vi "CR-字符检测参数读取.vi"(7 "error in (no error)":errorcluster caption="错误输入（无错误）", 10 "基路径":path) -> (0 "error out":errorcluster caption="错误输出", 1 "字符识别参数":T5={"Parameters (OCR/OCV 1)"={"Threshold Data"={"Method"=enum."Local", "Looking for"=1, "Color Mode"=0, "Kernel Size"={"Width"=32, "Height"=32}, "Ranges"=[{"Min"=1, "Max"=255}]}, "Reject Border"=TRUE, "Number Of Erosions"=0, "Size & Spacing"={"Segment Algorithm"=0, "Min Bounding Rect Width"=1, "Max Bounding Rect Width"=65536, "Min Bounding Rect Height"=1, "Max Bounding Rect Height"=65536, "Min Character Size"=20, "Max Character Size"=65536, "Min Char Spacing"=1, "Max Horiz Element Spacing"=1, "Max Vert Element Spacing"=0, "Max Space Distance"=65536}, "Read Options"={"Read Strategy"=1, "Read Resolution"=2, "Scale Dependant"=FALSE, "Aspect Ratio"=400, "Acceptance Level"=700, "Substitution Character"="?", "MultiLine"=TRUE}, "Valid Characters"=[], "Use Text Pattern"=FALSE, "Orientation"=0, "# Lines Expected"=0, "Number of Blocks"=4}, "Rectangle"={"Left"=0, "Top"=0, "Right"=0, "Bottom"=0, "Rotation"=0.0}, "字符长度判定"=0.0, "Reference System"={"Origin"={"X"=1245.2058, "Y"=1038.7815}, "Angle (deg)"=0.021420227, "Axis Reference"=0}, "File Path (字符库)"=path "D:/Inspect System/Source Code/Template Program/字符模板.abc", "File Path (连接件模板)"=path "D:/Inspect System/Source Code/Template Program/字符检测定位模板.png", "Url"="http://10.6.1.31:8080/MesInnerpackLineIO.asmx", "accessKey"="a45b2d3334ffs_\na45b2d3334ffs_"} {"Reference System"."Axis Reference" items=["Direct", "Indirect"]; "Rectangle"."Rotation" min=-90.0 max=90.0 step=1.0 format="%.2f"; "Rectangle"."Left" scale=0.0..1024.0; "Rectangle"."Right" scale=0.0..1024.0; "Parameters (OCR/OCV 1)"."Threshold Data"."Looking for" items=["Light on Dark", "Dark on Light"]; "Parameters (OCR/OCV 1)"."Threshold Data"."Color Mode" items=["RGB", "HSL", "HSV", "HSI"]; "Parameters (OCR/OCV 1)"."Size & Spacing"."Segment Algorithm" items=["None", "Shortest Segment", "Legacy Auto Split"]; "Parameters (OCR/OCV 1)"."Read Options"."Read Strategy" items=["Aggressive", "Conservative"]; "Parameters (OCR/OCV 1)"."Read Options"."Read Resolution" items=["Low", "Medium", "High"]; "Parameters (OCR/OCV 1)"."Valid Characters"."Pre-defined characters" items=["Any Character", "User-defined Characters", "Alphabetic", "Alphanumeric", "Uppercase Letters", "Lowercase Letters", "Decimal Digits", "Hexadecimal Digits", "Pattern", "Force Space"]; "Parameters (OCR/OCV 1)"."Orientation" items=["Baseline inside", "Baseline outside"]}, 2 "字符检测基础参数":T6={"IsNorImage"=TRUE, "Exposure Values"=100289, "ImagePath"=path "C:/Users/hedongpo/Desktop/514-hdp/Alignment Assemble System/Test Picture/B/3.bmp"} caption="参数界面" {"Exposure Values" scale=0.0..200000.0}, 3 "CR-CCD1字符定位参数":T4={"Rectangle"={"Left"=0, "Top"=0, "Right"=0, "Bottom"=0, "Rotation"=0.0}, "Settings"={"Curve Parameters"={"Extraction Mode"=0, "Edge Threshold"=35, "Edge Filter Size"=1, "Min Length"=25, "Row Search Step Size"=15, "Col Search Step Size"=15, "Max Endpoint Gap"=10, "Closed"=FALSE, "Subpixel"=FALSE}, "Match Mode"={"Rotation"=TRUE, "Scale"=FALSE, "Occlusion"=TRUE, "Reserved 1"=FALSE, "Reserved 2"=FALSE, "Reserved 3"=FALSE}, "Range Settings"=[{"Match Constraints"=0, "Min"=-17.0, "Max"=17.0}, {"Match Constraints"=2, "Min"=0.0, "Max"=25.0}], "Number of Matches"=1, "Minimum Match Score"=400.0, "SubPixel Accuracy"=FALSE, "Adv. Geometric Match Options 2"=[{"Setup Data Item"=21, "Item Value"=0.0}, {"Setup Data Item"=22, "Item Value"=1.0}]}, "Template File Path"=path "F:/Inspect System -2/Source Code/Template Program/程序1/字符定位模板.png"} {"Settings"."Curve Parameters"."Extraction Mode" items=["Normal", "Uniform Regions"]; "Settings"."Curve Parameters"."Edge Filter Size" items=["Fine", "Normal", "Contour Tracing"]; "Settings"."Curve Parameters"."Max Endpoint Gap" min=0; "Settings"."Curve Parameters"."Col Search Step Size" min=1 max=255 step=1; "Settings"."Curve Parameters"."Row Search Step Size" min=1 max=255 step=1; "Settings"."Curve Parameters"."Min Length" min=0; "Settings"."Curve Parameters"."Edge Threshold" min=1 max=350 step=1; "Settings"."Range Settings"."Max" format="%.2f"; "Settings"."Range Settings"."Min" format="%.2f"; "Settings"."Range Settings"."Match Constraints" items=["Rotation Angle (degrees)", "Scale Factor (%)", "Occlusion (%)"]; "Settings"."Adv. Geometric Match Options 2"."Setup Data Item" items=["Curve Extraction Mode", "Curve Edge Threshold", "Curve Edge Filter Size", "Min Curve Length", "Curve Row Search Step Size", "Curve Col Search Step Size", "Curve Max Endpoint Gap", "Extract Closed Curves", "Enable Subpixel Curve Extraction", "Enable Correlation Score", "Enable Subpixel Accuracy", "Subpixel Iterations", "Subpixel Tolerance", "Initial Match List Length", "Enable Target Template Curve Score", "Min Match Separation Distance", "Min Match Separation Angle", "Min Match Separation Scale", "Max Match Overlap", "Enable Coarse Result", "Enable Calibration Support", "Enable Contrast Reversal", "Search Strategy", "Refinement Match Factor", "Subpixel Match Factor"]; "Rectangle"."Rotation" format="%.2f"; "Rectangle"."Left" scale=0.0..1024.0; "Rectangle"."Right" scale=0.0..1024.0})   [LabVIEW 2017]
uses:
  <vilib>/vision/Pattern Matching.llb/IMAQ Curve Parameters.ctl
  <vilib>/vision/Pattern Matching.llb/IMAQ Match Range Setting.ctl
  <vilib>/Utility/xml.llb/Read From XML File(string).vi
  Global System.vi
panel:
  # "UI电源线反面标签1基础参数"
  # "D:\\Inspect System\\Source Code\\Template Program\\BlackTemplete"
  # "Range"
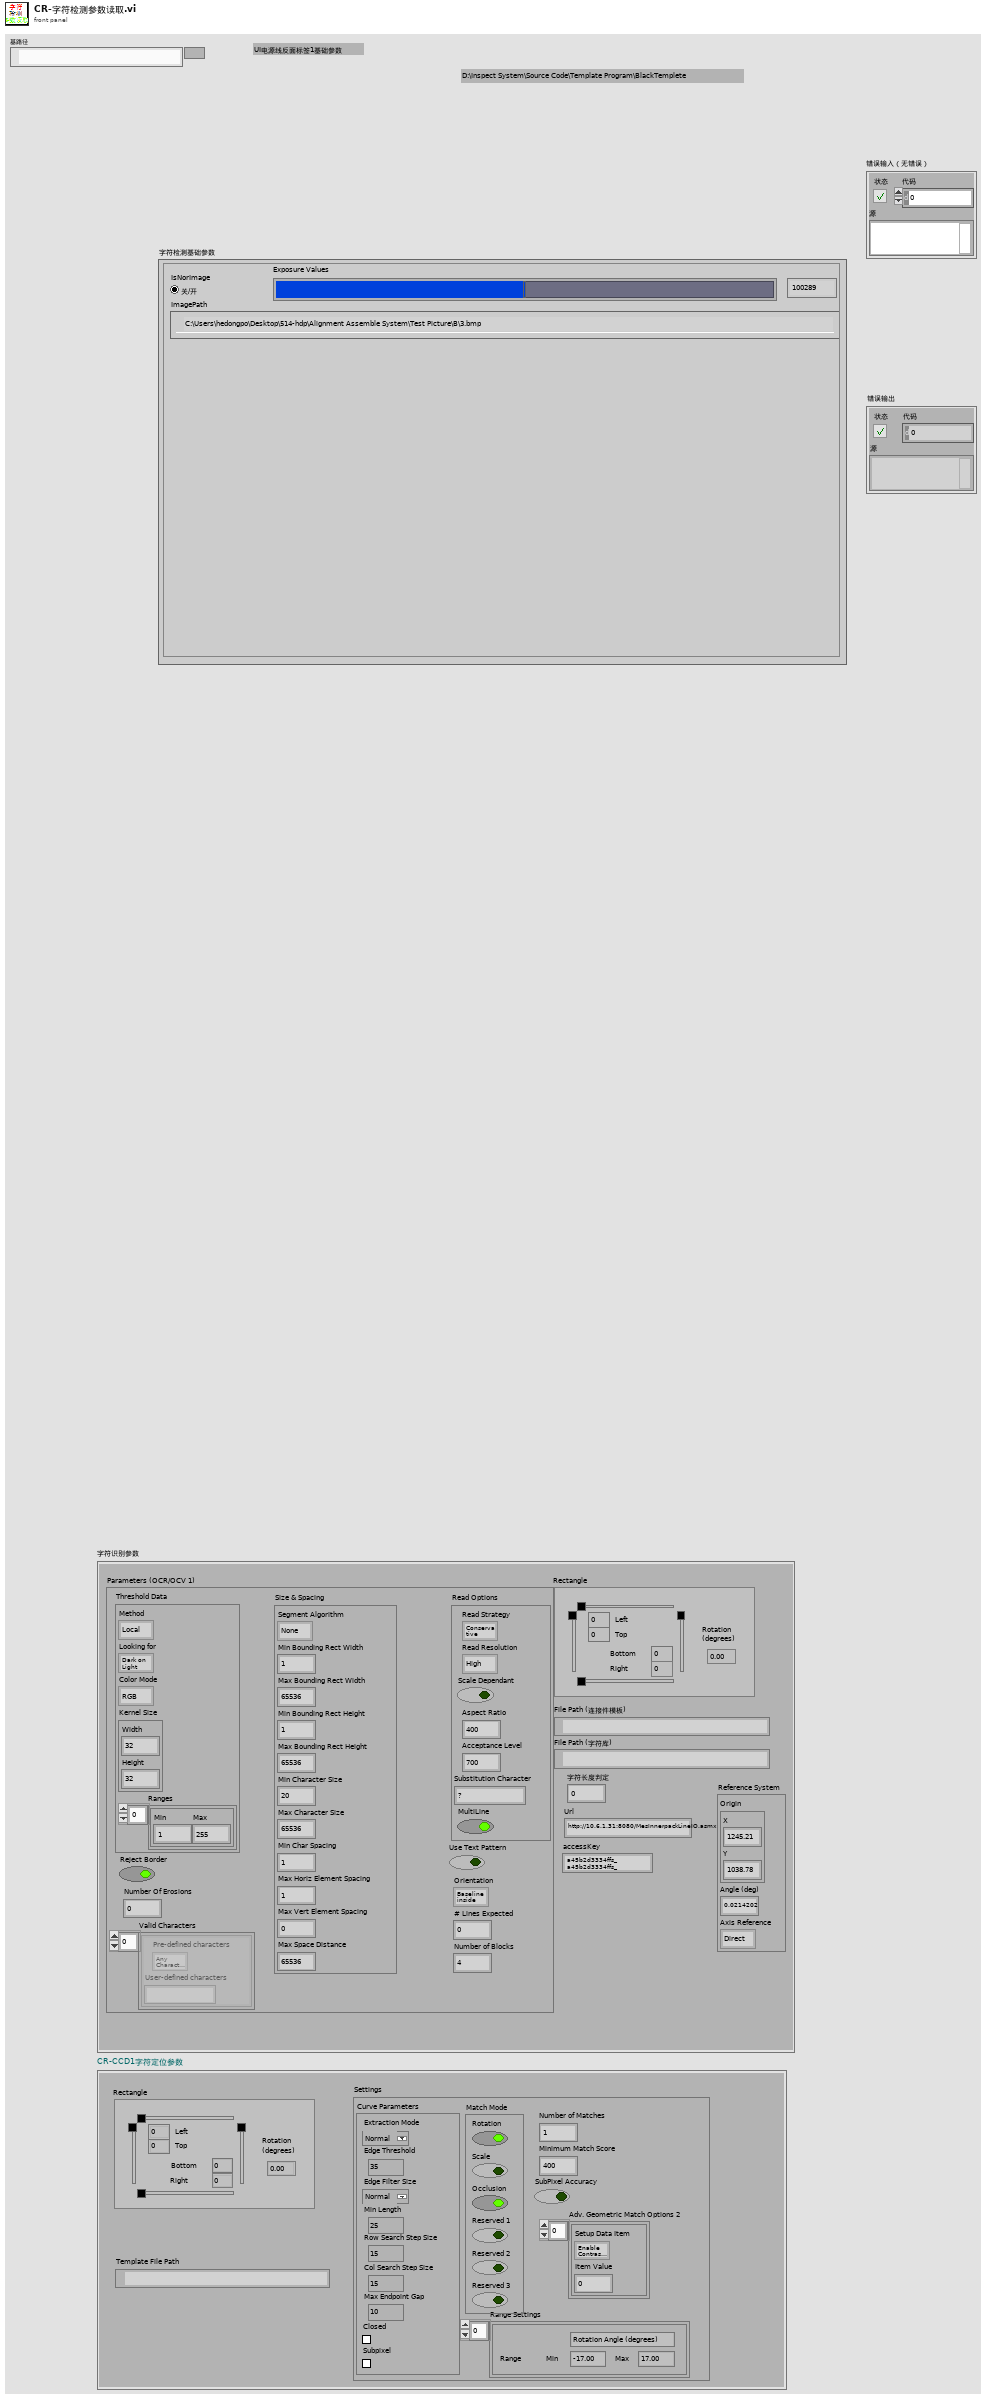
[diagram p1: front panel]
types:
  T1 = typedef "IMAQ Rectangle" = cluster{"Left":i32, "Top":i32, "Right":i32, "Bottom":i32, "Rotation":dbl}
  T2 = typedef "IMAQ Curve Parameters.ctl" = cluster{"Extraction Mode":u32, "Edge Threshold":i32, "Edge Filter Size":u32, "Min Length":i32, "Row Search Step Size":i32, "Col Search Step Size":i32, "Max Endpoint Gap":i32, "Closed":bool, "Subpixel":bool}
  T3 = typedef "IMAQ Match Range Setting.ctl" = cluster{"Match Constraints":u32, "Min":dbl, "Max":dbl}
  T4 = cluster{"Rectangle":T1, "Settings":cluster{"Curve Parameters":T2, "Match Mode":cluster{"Rotation":bool, "Scale":bool, "Occlusion":bool, "Reserved 1":bool, "Reserved 2":bool, "Reserved 3":bool}, "Range Settings":T3[], "Number of Matches":i32, "Minimum Match Score":sgl, "SubPixel Accuracy":bool, "Adv. Geometric Match Options 2":cluster{"Setup Data Item":u16, "Item Value":dbl}[]}, "Template File Path":path}
  T5 = cluster{"Parameters (OCR/OCV 1)":cluster{"Threshold Data":cluster{"Method":enum16{"Fixed Range", "Uniform", "Linear", "Non Linear", "Local", "Color"}, "Looking for":u32, "Color Mode":u32, "Kernel Size":cluster{"Width":i32, "Height":i32}, "Ranges":cluster{"Min":i32, "Max":i32}[]}, "Reject Border":bool, "Number Of Erosions":i32, "Size & Spacing":cluster{"Segment Algorithm":u16, "Min Bounding Rect Width":i32, "Max Bounding Rect Width":i32, "Min Bounding Rect Height":i32, "Max Bounding Rect Height":i32, "Min Character Size":i32, "Max Character Size":i32, "Min Char Spacing":i32, "Max Horiz Element Spacing":i32, "Max Vert Element Spacing":i32, "Max Space Distance":i32}, "Read Options":cluster{"Read Strategy":i32, "Read Resolution":i32, "Scale Dependant":bool, "Aspect Ratio":i32, "Acceptance Level":i32, "Substitution Character":string, "MultiLine":bool}, "Valid Characters":cluster{"Pre-defined characters":i32, "User-defined characters":string}[], "Use Text Pattern":bool, "Orientation":u32, "# Lines Expected":u32, "Number of Blocks":i32}, "Rectangle":T1, "字符长度判定":dbl, "Reference System":cluster{"Origin":cluster{"X":sgl, "Y":sgl}, "Angle (deg)":sgl, "Axis Reference":u32}, "File Path (字符库)":path, "File Path (连接件模板)":path, "Url":string, "accessKey":string}
  T6 = cluster{"IsNorImage":bool, "Exposure Values":u32, "ImagePath":path}
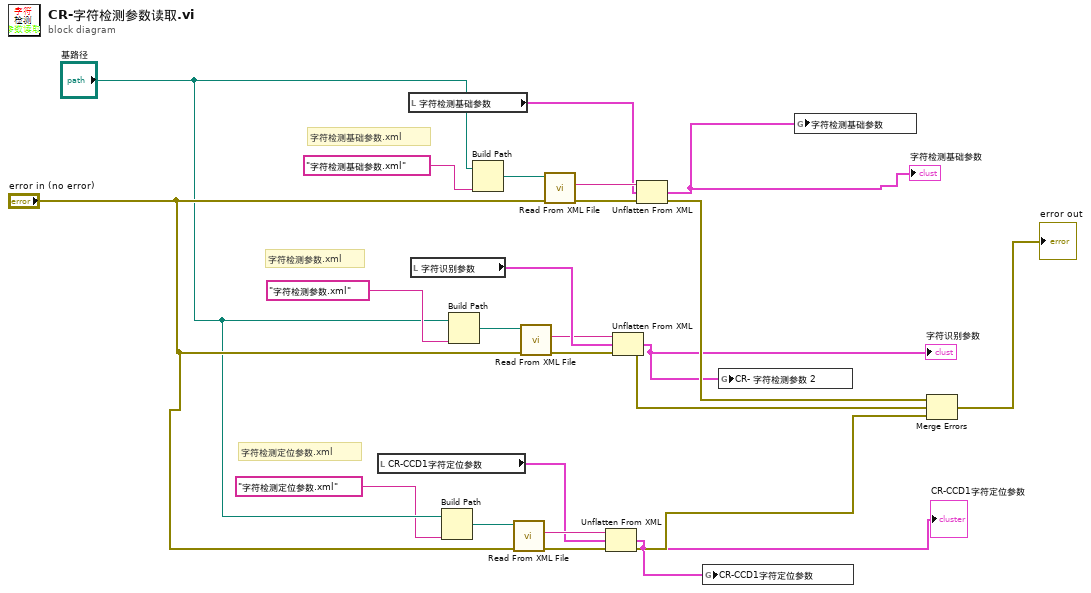
[diagram p0: block diagram]
diagram:
  # "字符检测定位参数.xml"
  # "字符检测参数.xml"
  # "字符检测基础参数.xml"
  n1 = local read "CR-CCD1字符定位参数"() -> (w1:T4)
  n2 = local read "字符检测基础参数"() -> (w21:T6)
  n3 = local read "字符识别参数"() -> (w15:T5)
  n4 = Build Path(base path="基路径", name or relative path="字符检测定位参数.xml" ("名称或相对路径")) -> (appended path=w3:path)
  n5 = Build Path(base path="基路径", name or relative path="字符检测参数.xml" ("名称或相对路径")) -> (appended path=w13:path)
  n6 = Build Path(base path="基路径", name or relative path="字符检测基础参数.xml" ("名称或相对路径")) -> (appended path=w23:path)
  n7 = call-poly <vilib>:"Read From XML File.vi"("error in (no error)"="error in (no error)", "XML File Path"=w3) -> ("error out"=w4:errorcluster, "XML Elements"=w2:string)  [unwired: 7 in, 1 out]
  n8 = call-poly <vilib>:"Read From XML File.vi"("error in (no error)"="error in (no error)", "XML File Path"=w13) -> ("error out"=w12:errorcluster, "XML Elements"=w14:string)  [unwired: 7 in, 1 out]
  n9 = call-poly <vilib>:"Read From XML File.vi"("error in (no error)"="error in (no error)", "XML File Path"=w23) -> ("error out"=w20:errorcluster, "XML Elements"=w22:string)  [unwired: 7 in, 1 out]
  n10 = Unflatten From XML(xml string=w2, type=w1, error in (no error)=w4) -> (value=w6:T4, error out=w9:errorcluster)
  "CR-CCD1字符定位参数" <- w6
  n11 = Unflatten From XML(xml string=w14, type=w15, error in (no error)=w12) -> (value=w10:T5, error out=w16:errorcluster)
  "字符识别参数" <- w10
  n12 = Unflatten From XML(xml string=w22, type=w21, error in (no error)=w20) -> (value=w17:T6, error out=w19:errorcluster)
  "字符检测基础参数" <- w17
  n13 = global write "Global System.vi" "CR-CCD1字符定位参数"(w6) -> ()
  n14 = global write "Global System.vi" "CR- 字符检测参数 2"(w10) -> ()
  n15 = global write "Global System.vi" "字符检测基础参数"(w17) -> ()
  n16 = Merge Errors(w19, w16, w9) -> (→"error out":errorcluster)
